vi "ADXL345_Read.vi"(3 "error in":errorcluster, 6 "Arduino Resource":T2={"VISA resource"="", "Board Type"=enum."Uno", "Connection Type"=enum."USB / Serial", "Bytes Per Packet (15)"=15}) -> (0 "error out":errorcluster, 1 "Raw Accelerometer Data":T1, 2 "Arduino Resource":T2={"VISA resource"="", "Board Type"=enum."Uno", "Connection Type"=enum."USB / Serial", "Bytes Per Packet (15)"=15})   [LabVIEW 2012]
uses:
  <vilib>/LabVIEW Interface for Arduino/Type Defs/Arduino Resource.ctl
  <vilib>/LabVIEW Interface for Arduino/Type Defs/Board Type.ctl
  <vilib>/LabVIEW Interface for Arduino/LabVIEW Interface for Arduino.lvlib
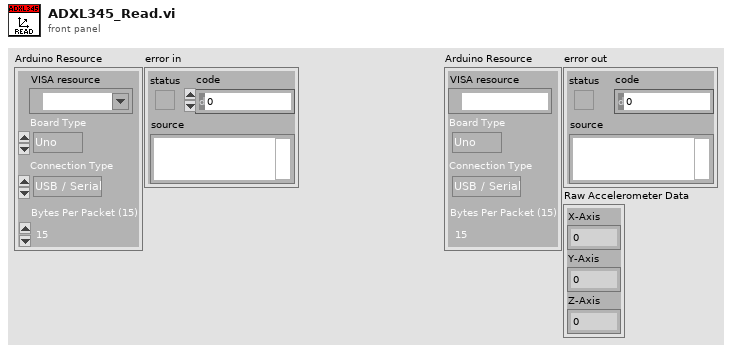
[diagram p1: front panel]
types:
  T1 = cluster{"X-Axis":i32, "Y-Axis":i32, "Z-Axis":i32}
  T2 = typedef "LabVIEW Interface for Arduino.lvlib/Arduino Resource.ctl" = cluster{"VISA resource":refnum<visa-resource-name>, "Board Type":T3, "Connection Type":enum8{"USB / Serial"}, "Bytes Per Packet (15)":u8}
  T3 = typedef "LabVIEW Interface for Arduino.lvlib/Board Type.ctl" = enum16{"Uno", "Dimuelanove w/Atmega 328", "Mega 2560"}
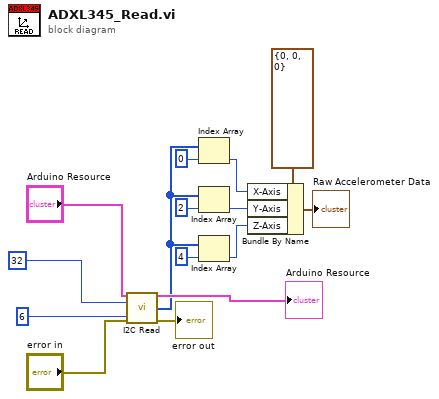
[diagram p0: block diagram]
diagram:
  n1 = call <vilib>:"I2C Read.vi"("Arduino Resource"="Arduino Resource", "Address (0)"=u8 32 ("Address (0x32)"), "Bytes To Read"=u8 6 ("Bytes To Read (6)"), "error in"="error in") -> ("Arduino Resource"=→"Arduino Resource":T2, "I2C Data"=w9:u8[], "error out"=→"error out":errorcluster)  [unwired: 9 in]
  n2 = Index Array(array=w9, index=0) -> (element=w5:u8)
  n3 = Index Array(array=w9, index=2) -> (element=w4:u8)
  n4 = Index Array(array=w9, index=4) -> (element=w3:u8)
  n5 = Bundle By Name(cluster=T1 {"X-Axis"=0, "Y-Axis"=0, "Z-Axis"=0} ("input cluster"), "X-Axis"=w5, "Y-Axis"=w4, "Z-Axis"=w3) -> (→"Raw Accelerometer Data":T1)
